vi "(SubVI) Deal with Delay between Scan and Record From Stage Array.vi"(4 "Avg. time delay (ms)":dbl=18.0, 5 "Toward first ?\nT=+, F=-":bool, 6 "Record scan rate  (um/s)":dbl=2.0 format="%.3f", 7 "Real initial position (um)":dbl format="%0.5f", 8 "Folded Stage Array (um)":dbl[](array[numeric]), 9 "Unfolded Stage Array (um)":dbl[](array[numeric])) -> (0 "Stage Array Shift (um)":dbl, 2 "Correct Folded Stage Array (um)":dbl[](array[numeric]), 3 "Correct Unfolded Stage Array (um)":dbl[](array[numeric]))   [LabVIEW 2014]
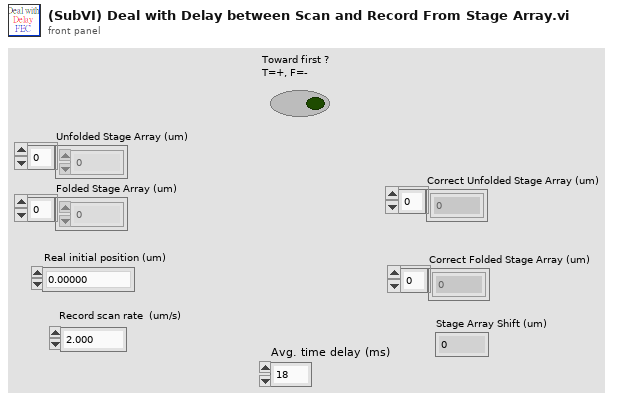
[diagram p1: front panel]
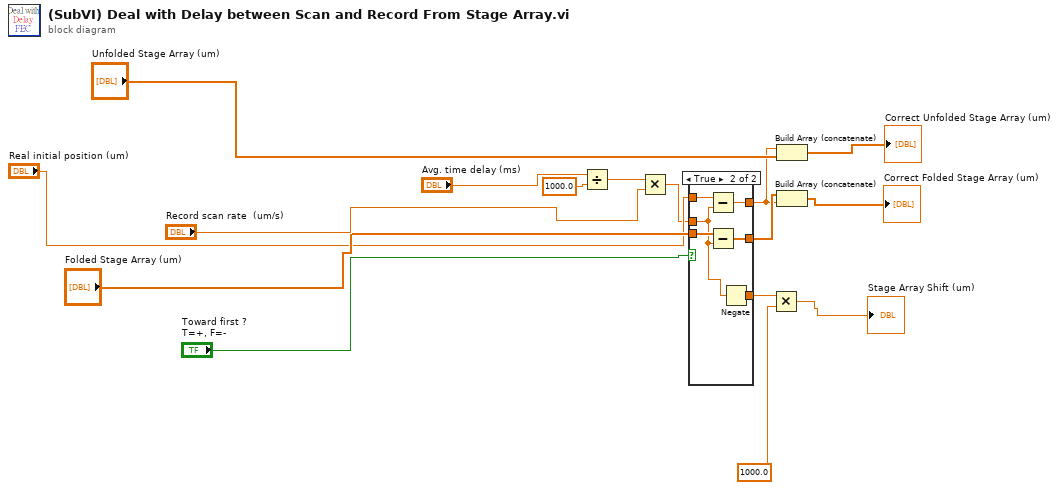
[diagram p0: block diagram]
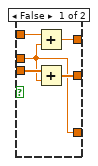
[diagram p2: hidden frame]
diagram:
  n1 = Divide(x="Avg. time delay (ms)", y=1000.0) -> (x/y=w9:dbl)
  n2 = Multiply(x=w9, y="Record scan rate  (um/s)") -> (x*y=w11:dbl)
  n3 = case shown="True" "Toward first ?\nT=+, F=-" {
    tunnel: "Folded Stage Array (um)" -> [w21 w27]
    tunnel: w11 -> [w17 w23]
    tunnel: [w20 w26] -> w7
    tunnel: "Real initial position (um)" -> [w19 w25]
    tunnel: [w18 w24] -> w6
    tunnel: [w17 w22] -> w3
    frame False {
      n4 = Add(x=w19, y=w17) -> (x+y=w18:dbl)
      n5 = Add(x=w21, y=w17) -> (x+y=w20:dbl[])
    }
    frame True {
      n6 = Subtract(x=w25, y=w23) -> (x-y=w24:dbl)
      n7 = Subtract(x=w27, y=w23) -> (x-y=w26:dbl[])
      n8 = Negate(x=w23) -> (-x=w22:dbl)
    }
  }
  n9 = Multiply(x=w3, y=1000.0) -> (x*y=→"Stage Array Shift (um)":dbl)
  n10 = Build Array (concatenate)(w6, "Unfolded Stage Array (um)") -> (→"Correct Unfolded Stage Array (um)":dbl[])
  n11 = Build Array (concatenate)(w7, w6) -> (→"Correct Folded Stage Array (um)":dbl[])
